vi "Robot Global Data.vi"() -> ()   [LabVIEW 2015]
doc: "This global VI can contain as many global variables as you need. Place a control on the panel, give it a good name. To read or write to it from a VI, drag the icon to the diagram of that VI. You can also drag from the project. Click on the node to change which global you access. You shouldn't have multiple locations writing to a global or it will cause a race-condition."
uses:
  <vilib>/Rock Robotics/WPI/Camera/WPI_CameraImageSize.ctl
  <vilib>/Rock Robotics/WPI/DriverStation/WPI_DriverStationRobotMode2.ctl
panel:
  in  "Goal Info":cluster{"Angle":dbl, "RPM":dbl}
  in  "Defenses Enum":T1(ring)
  in  "Current X/Y":cluster{"X":dbl, "Y":dbl}
  in  "Defense Offset":dbl[](array[numeric])
  in  "Defense Dist":dbl[](array[numeric])
  in  "Robot Mode":T2
  in  "image size":T3=enum."320x240"
  in  "Enable Vision":bool
  # "Distance from defense ramp and horizontal offset"
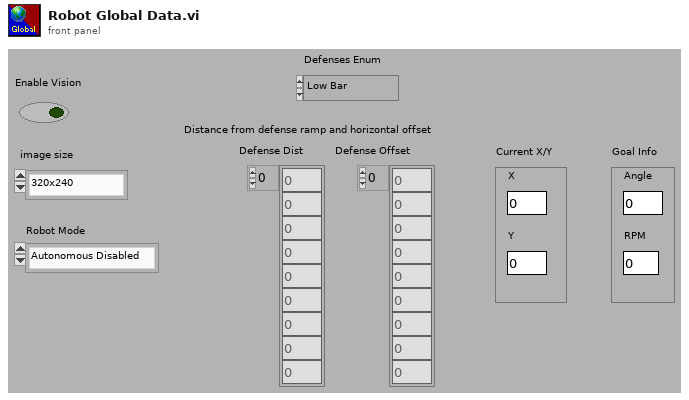
[diagram p1: front panel]
types:
  T1 = enum8{"Low Bar", "Porticullis", "Cheval de Frise", "Moat", "Ramparts", "Drawbridge", "Sally Port", "Rock Wall", "Rough Terrain"}
  T2 = typedef "WPI_DriverStationRobotMode2.ctl" = enum16{"Autonomous Disabled", "Autonomous Enabled", "Teleop Disabled", "Teleop Enabled", "Disconnected", "Finish", "Test Disabled", "Test Enabled", "Emergency Stopped"}
  T3 = typedef "WPI_CameraImageSize.ctl" = enum16{"640x480", "320x240", "160x120", "Custom"}
diagram:
